vi "regSubEvents.vi"(8 "error in (no error)":errorcluster, 11 "SALCommunicator in":refnum<class "SALCommunicatorDL.lvclass">) -> (0 "error out":errorcluster, 2 "Event Registration Refnum":refnum<event-registration>, 3 "SALCommunicator out":refnum<class "SALCommunicatorDL.lvclass">)   [LabVIEW 2016, in "SALCommunicatorDL.lvclass"]
uses:
  SALCommunicatorDL.lvclass
  <vilib>/Utility/error.llb/DialogType.ctl
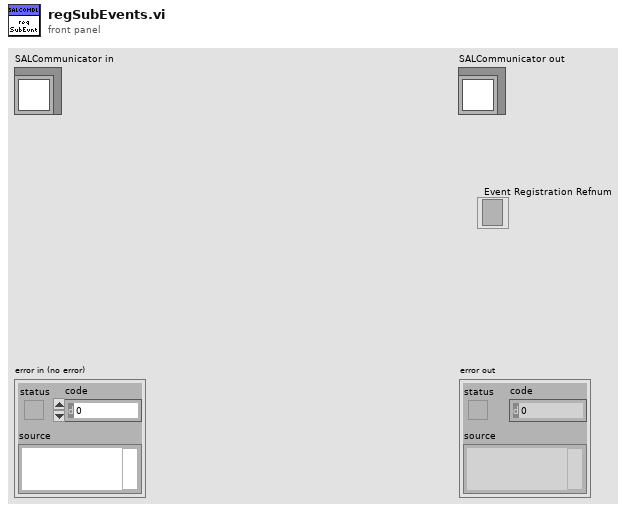
[diagram p1: front panel]
types:
  T1 = typedef "DialogType.ctl" = u16
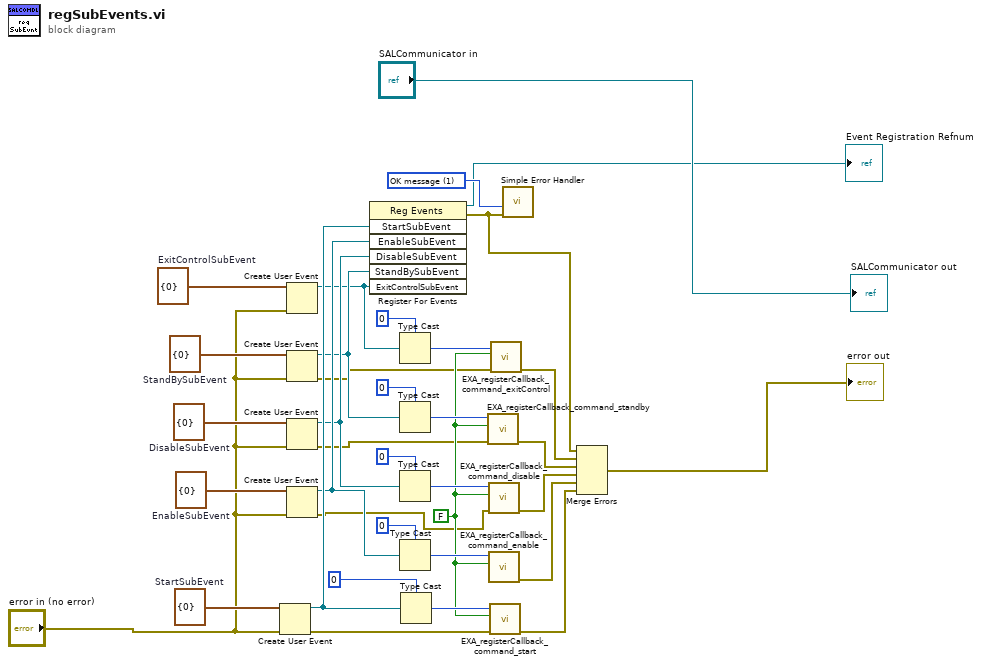
[diagram p0: block diagram]
diagram:
  w22 = cluster{"Data":i32} {"Data"=0}  # ExitControlSubEvent
  w24 = cluster{"Data":i32} {"Data"=0}  # StandBySubEvent
  w29 = cluster{"Data":i32} {"Data"=0}  # DisableSubEvent
  w32 = cluster{"Data":i32} {"Data"=0}  # EnableSubEvent
  w35 = cluster{"Data":i32} {"Data"=0}  # StartSubEvent
  w36 = T1 1 items=["no dialog", "OK message", "continue or stop message", "OK message + warnings", "continue/stop + warnings"] ("type of dialog (OK msg:1)")
  w15 = FALSE ("skipOld")
  n1 = Create User Event(user event datatype=w35, error in="error in (no error)") -> (user event=w33:refnum<user-event>, error out=w14:errorcluster)
  n2 = Create User Event(user event datatype=w22, error in="error in (no error)") -> (user event=w21:refnum<user-event>)  [unwired: 1 out]
  n3 = Create User Event(user event datatype=w24, error in="error in (no error)") -> (user event=w25:refnum<user-event>, error out=w11:errorcluster)
  n4 = Create User Event(user event datatype=w29, error in="error in (no error)") -> (user event=w27:refnum<user-event>, error out=w12:errorcluster)
  n5 = Create User Event(user event datatype=w32, error in="error in (no error)") -> (user event=w30:refnum<user-event>, error out=w13:errorcluster)
  n6 = register-events(w33, w30, w27, w25, w21) -> (reference out=→"Event Registration Refnum":refnum<event-registration>, error out=w5:errorcluster)  [unwired: 2 in]
  n7 = Type Cast(type=0, x=w21) -> (*(type *) &x=w16:i32)
  n8 = Type Cast(type=0, x=w25) -> (*(type *) &x=w17:i32)
  n9 = Type Cast(type=0, x=w27) -> (*(type *) &x=w18:i32)
  n10 = Type Cast(type=0, x=w30) -> (*(type *) &x=w19:i32)
  n11 = Type Cast(type=0, x=w33) -> (*(type *) &x=w20:i32)
  n12 = call "EXA_registerCallback_command_standby.vi"("error in (no error)"=w12, "skipOld"=w15, "handle"=w17) -> ("error out"=w9:errorcluster)  [unwired: 7 in, 1 out]
  n13 = call "EXA_registerCallback_command_disable.vi"("error in (no error)"=w13, "skipOld"=w15, "handle"=w18) -> ("error out"=w8:errorcluster)  [unwired: 7 in, 1 out]
  n14 = call "EXA_registerCallback_command_enable.vi"("skipOld"=w15, "handle"=w19) -> ("error out"=w7:errorcluster)  [unwired: 8 in, 1 out]
  n15 = call "EXA_registerCallback_command_start.vi"("error in (no error)"=w14, "skipOld"=w15, "handle"=w20) -> ("error out"=w6:errorcluster)  [unwired: 7 in, 1 out]
  n16 = call "EXA_registerCallback_command_exitControl.vi"("error in (no error)"=w11, "skipOld"=w15, "handle"=w16) -> ("error out"=w10:errorcluster)  [unwired: 7 in, 1 out]
  n17 = call <vilib>:"Simple Error Handler.vi"("type of dialog (OK msg:1)"=w36, "error in (no error)"=w5) -> ()  [unwired: 3 in, 5 out]
  n18 = Merge Errors(w5, w10, w9, w8, w7, w6) -> (→"error out":errorcluster)
  "SALCommunicator out" <- "SALCommunicator in"
